vi "INBETRIEBNAHME AVL GNU63.vi"() -> ()   [LabVIEW 2015, in "Linearisierung v2.lvlib" / "Gasteiler.lvlib" / "AK Komm Gasteiler.lvlib"]
uses:
  AK Komm Gasteiler.lvlib
panel:
  in  "OK-Schaltfläche":bool
  in  "Port":u16
  in  "Adresse":string
  in  "löschen":bool
  out "Daten":string
  out "Befehl (Antwort)":string
  out "Empfangsdaten":string[](array[string])
  out "ES (Error Status)":string
  in  "Sendedaten":string[](array[string])
  in  "Kanalnummer (0)":u8
  in  "Befehl (4 Zeichen)":string="STBY"
  out "error out":errorcluster caption="Fehler (Ausgang)"
  in  "ausführen":bool
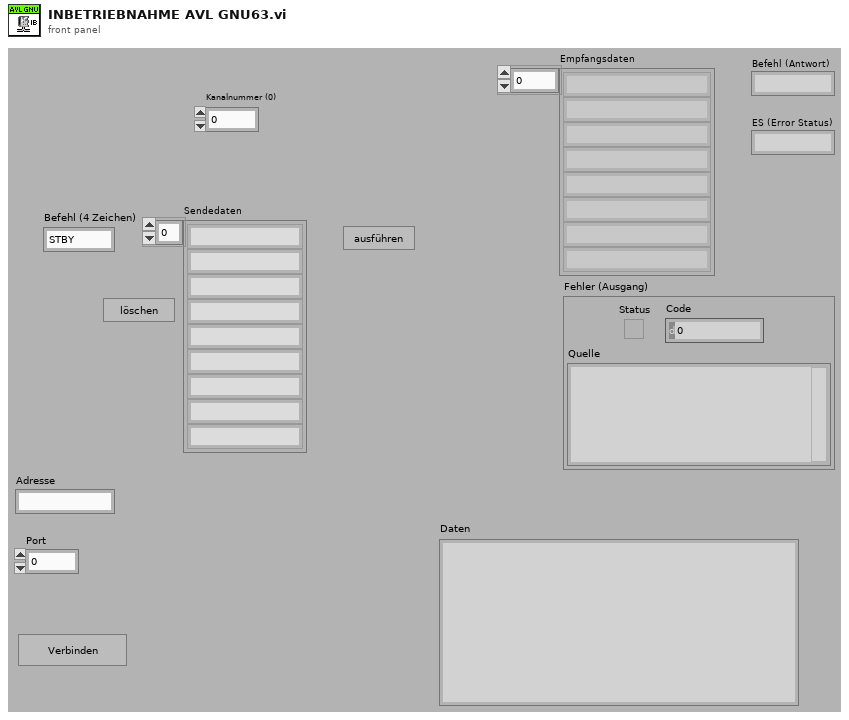
[diagram p1: front panel]
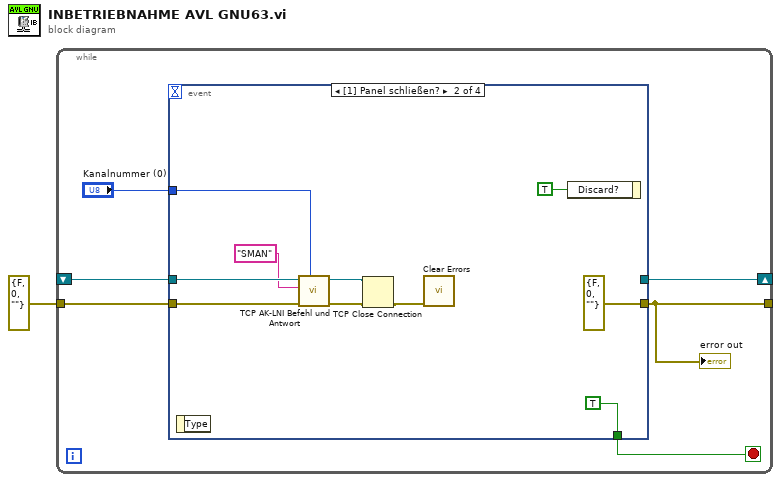
[diagram p0: block diagram]
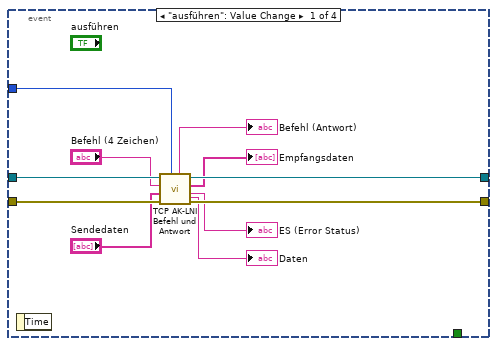
[diagram p2: hidden frame]
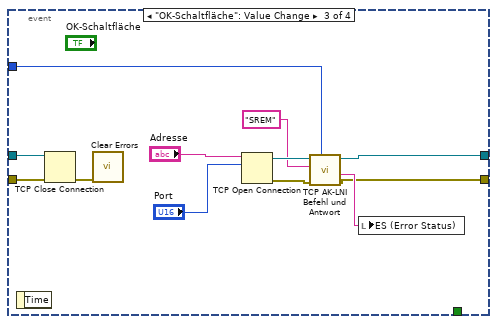
[diagram p3: hidden frame]
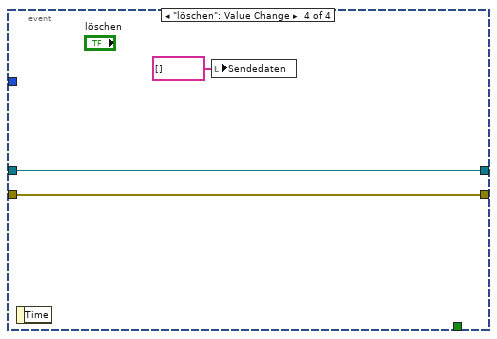
[diagram p4: hidden frame]
diagram:
  n1 = while {
    shift-right: [w5] -> _
    shift-left: _ -> [w7]
    tunnel: errorcluster {"status"=FALSE, "code"=0, "source"=""} ("Fehler (Eingang, kein Fehler)") -> [w6]
    tunnel: [w2] -> _
    stop <- w4 stop-if-true
    n2 = event shown="[1] Panel schließen?" {
      selector: _ -> [_ _ _ _]
      dyn-events: _ -> [_ _ _ _]
      timeout: _ -> [_ _ _ _]
      tunnel: w7 -> [w18 w25 w40 w43]
      tunnel: w6 -> [w17 w24 w39 w42]
      tunnel: [w16 _ w31 w43] -> w5
      tunnel: [w15 errorcluster {"status"=FALSE, "code"=0, "source"=""} ("Fehler (Ausgang)") w29 w42] -> w2
      tunnel: [_ TRUE _ _] -> w4
      tunnel: "Kanalnummer (0)" -> [w13 w23 w32 _]
      event "ausführen": Value Change {
        n3 = event-data() -> ()  [unwired: 1 in, 1 out]
        n4 = call "TCP AK-LNI Befehl und Antwort.vi"("Kanalnummer (0)"=w13, "Fehler (Eingang)"=w17, "Sendedaten"="Sendedaten", "Befehl (4 Zeichen)"="Befehl (4 Zeichen)", "Verbindungs-ID"=w18) -> ("Fehler (Ausgang)"=w15:errorcluster, "ES (Error Status)"=→"ES (Error Status)":string, "Empfangsdaten"=→"Empfangsdaten":string[], "Verbindungs-ID"=w16:refnum<k5>, "Daten"=→"Daten":string, "Befehl (Antwort)"=→"Befehl (Antwort)":string)  [unwired: 1 in]
      }
      event Panel Close? {
        n5 = event-data() -> ()  [unwired: 1 in, 1 out]
        n6 = call "TCP AK-LNI Befehl und Antwort.vi"("Kanalnummer (0)"=w23, "Fehler (Eingang)"=w24, "Befehl (4 Zeichen)"="SMAN", "Verbindungs-ID"=w25) -> ("Fehler (Ausgang)"=w20:errorcluster, "Verbindungs-ID"=w21:refnum<k5>)  [unwired: 2 in, 4 out]
        n7 = TCP Close Connection(connection ID=w21, error in (no error)=w20) -> (error out=w19:errorcluster)  [unwired: 1 in, 1 out]
        n8 = call <vilib>:"Clear Errors.vi"("error in (no error)"=w19) -> ()  [unwired: 5 in, 2 out]
        n9 = event-data("Discard?"=TRUE ("Verwerfen?")) -> ()  [unwired: 1 in, 1 out]
      }
      event "OK-Schaltfläche": Value Change {
        n10 = event-data() -> ()  [unwired: 1 in, 1 out]
        n11 = TCP Close Connection(connection ID=w40, error in (no error)=w39) -> (error out=w38:errorcluster)  [unwired: 1 in, 1 out]
        n12 = call <vilib>:"Clear Errors.vi"("error in (no error)"=w38) -> ()  [unwired: 5 in, 2 out]
        n13 = TCP Open Connection(address="Adresse", remote port or service name="Port") -> (connection ID=w35:refnum<k5>, error out=w33:errorcluster)  [unwired: 3 in]
        n14 = call "TCP AK-LNI Befehl und Antwort.vi"("Kanalnummer (0)"=w32, "Fehler (Eingang)"=w33, "Befehl (4 Zeichen)"="SREM", "Verbindungs-ID"=w35) -> ("Fehler (Ausgang)"=w29:errorcluster, "ES (Error Status)"=w30:string, "Verbindungs-ID"=w31:refnum<k5>)  [unwired: 2 in, 3 out]
        n15 = local write "ES (Error Status)"(w30) -> ()
      }
      event "löschen": Value Change {
        n16 = event-data() -> ()  [unwired: 1 in, 1 out]
        n17 = local write "Sendedaten"(string[] [] ("Sendedaten")) -> ()
      }
    }
    "error out" <- w2
  }
